vi "read_params.vi"(8 "error in (no error)":errorcluster caption="entrée d'erreur (pas d'erreur)", 11 "FactorAnalysis en entrée":refnum<class "FactorAnalysis.lvclass">) -> (0 "error out":errorcluster caption="sortie d'erreur", 2 "params":T1={"n_components"={"n_components_type"="None", "n_components_int"=0.0}, "tol"=0.0, "copy"=TRUE, "max_iter"=0.0, "noise_variance_init"={"noise_variance_init_type"="None", "noise_variance_init_list"=[]}, "svd_method"="randomized", "iterated_power"=3.0, "rotation"="None", "random_state"=0.0}, 3 "FactorAnalysis en sortie":refnum<class "FactorAnalysis.lvclass">)   [LabVIEW 2020, in "FactorAnalysis.lvclass"]
uses:
  FactorAnalysis.lvclass
  Controls/factor_analysis_params.ctl
  FactorAnalysis.lvclass/FactorAnalysis.ctl
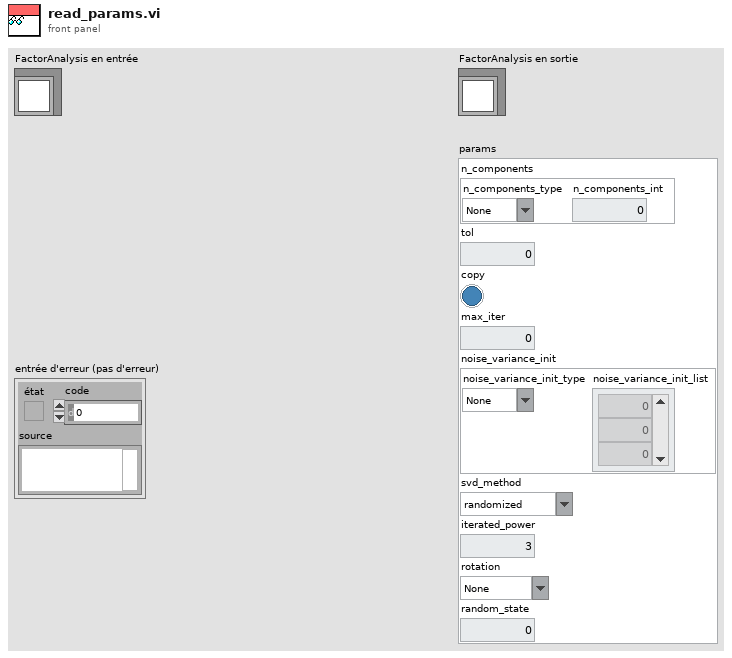
[diagram p1: front panel]
types:
  T1 = typedef "factor_analysis_params.ctl" = cluster{"n_components":cluster{"n_components_type":string, "n_components_int":dbl}, "tol":dbl, "copy":bool, "max_iter":dbl, "noise_variance_init":cluster{"noise_variance_init_type":string, "noise_variance_init_list":dbl[]}, "svd_method":string, "iterated_power":dbl, "rotation":string, "random_state":dbl}
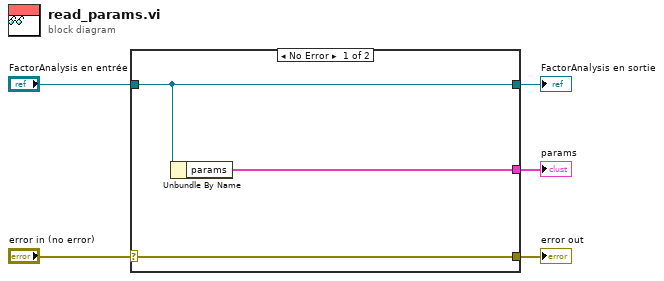
[diagram p0: block diagram]
diagram:
  n1 = case shown="No Error" "error in (no error)" {
    selector: "error in (no error)" -> [w8 w9]
    tunnel: [w8 w9] -> w4
    tunnel: [w7 w10] -> w2
    tunnel: "FactorAnalysis en entrée" -> [w7 w10]
    tunnel: [w6 _] -> w1
    frame No Error {
      n2 = Unbundle By Name(w7) -> ("params"=w6:T1)
    }
    frame Error {
    }
  }
  "error out" <- w4
  "FactorAnalysis en sortie" <- w2
  "params" <- w1
